vi "FPGA Acquire Loop.vi"(8 "error in (no error)":errorcluster, 10 "FIFO Buffers":refnum<k33>[](array[refnum]), 11 "Refnum in":refnum<k20>) -> ()   [LabVIEW 2014]
uses:
  Controls/RT Stream Data.ctl
  RT Stop.vi
  RT Tags.vi
  RT Comm Refs.vi
  <vilib>/Utility/error.llb/Error Cluster From Error Code.vi
  <vilib>/rvi/errors/niLvFpgaAdjustHostInterfaceError.vi
  <vilib>/rvi/interface/nirviMethod/nirviMethod.xnode
  <vilib>/rvi/interface/nirviReadWriteControl/nirviReadWriteControl.xnode
  <vilib>/FPGAPlugInAG/Dynamic/niLvFpga_ReadFifo_Dynamic.vi
  <vilib>/rvi/errors/niLvFpgaMergeErrorWithErrorCode.vi
  NiFpgaLv.dll
  <vilib>/rvi/interface/Simulation/niFpgaSimulationCallBeginRW.vi
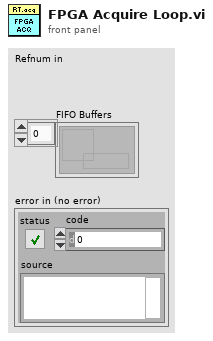
[diagram p1: front panel]
types:
  T1 = typedef "RT Stream Data.ctl" = cluster{"Temp Data":dbl[], "pH Data":dbl[]}
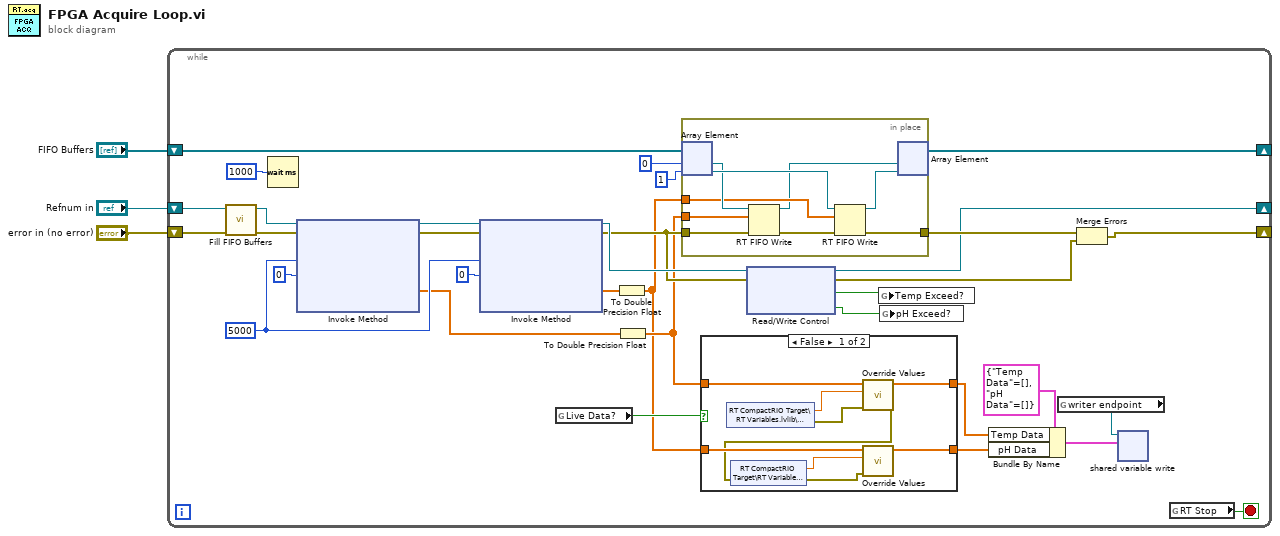
[diagram p0: block diagram]
diagram:
  n1 = while {
    shift-right: [w18] -> _
    shift-left: "Refnum in" -> [w36]
    shift-right: [w16] -> _
    shift-left: "error in (no error)" -> [w34]
    shift-right: [w21] -> _
    shift-left: "FIFO Buffers" -> [w26]
    stop <- w14 stop-if-true
    w30 = u32 5000 ("Number of Elements")
    n2 = call "Fill FIFO Buffers.vi"("error in (no error)"=w34, "Refnum in"=w36) -> ("error out"=w29:errorcluster, "Refnum out"=w33:refnum<k20>)  [unwired: 8 in]
    n3 = Wait (ms)(milliseconds to wait=u32 1000) -> ()  [unwired: 1 out]
    n4 = xnode "Invoke Method"("FPGA VI Reference In"=w33, "error in"=w29, "Number of Elements"=w30, "Timeout (ms)"=0) -> ("FPGA VI Reference Out"=w32:refnum<k20>, "error out"=w31:errorcluster, "Data"=w23:sgl[])  [unwired: 1 out]
    n5 = xnode "Invoke Method"("FPGA VI Reference In"=w32, "error in"=w31, "Number of Elements"=w30, "Timeout (ms)"=0) -> ("FPGA VI Reference Out"=w19:refnum<k20>, "error out"=w17:errorcluster, "Data"=w22:sgl[])  [unwired: 1 out]
    n6 = global read "RT Tags.vi" "Live Data?"() -> (w13:bool)
    n7 = To Double Precision Float(number=w22) -> (double precision float=w9:dbl[])
    n8 = To Double Precision Float(number=w23) -> (double precision float=w10:dbl[])
    n9 = in-place {
      in-place-border: w17 -> [w55]
      in-place-border: w10 -> [w52]
      in-place-border: w9 -> [w51]
      in-place-border: [w48] -> w20
      n10 = in-place-array #1(w26, 0, 1) -> (w53:refnum<k33>, w54:refnum<k33>)
      n11 = RT FIFO Write(0:w53, 1:w52, 3:w55) -> (8:w50:refnum<k33>, 11:w56:errorcluster)  [unwired: 2 in, 2 out]
      n12 = RT FIFO Write(0:w54, 1:w51, 3:w56) -> (8:w49:refnum<k33>, 11:w48:errorcluster)  [unwired: 2 in, 2 out]
      n13 = in-place-array #1(w50, w49) -> (w21:refnum<k33>[])  [unwired: 2 out]
    }
    n14 = case shown="False" w13 {
      tunnel: w10 -> [w45 w47]
      tunnel: w9 -> [w43 w46]
      tunnel: [w44 w47] -> w8
      tunnel: [w42 w46] -> w7
      frame False {
        n15 = shared-variable "RT CompactRIO Target\\RT Variables.lvlib\\TempOV"() -> (w41:dbl, error out=w39:errorcluster)  [unwired: 1 in]
        n16 = call "Override Values.vi"("error in (no error)"=w39, "Double"=w41, "Array in"=w45) -> ("error out"=w38:errorcluster, "Array out"=w44:dbl[])  [unwired: 7 in]
        n17 = shared-variable "RT CompactRIO Target\\RT Variables.lvlib\\pHOV"(error in=w38) -> (w40:dbl, error out=w37:errorcluster)
        n18 = call "Override Values.vi"("error in (no error)"=w37, "Double"=w40, "Array in"=w43) -> ("Array out"=w42:dbl[])  [unwired: 7 in, 1 out]
      }
      frame True {
      }
    }
    n19 = xnode "Read/Write Control"("FPGA VI Reference In"=w19, "error in"=w17) -> ("FPGA VI Reference Out"=w18:refnum<k20>, "error out"=w15:errorcluster, "Temp Exceed?"=w12:bool, "pH Exceed?"=w11:bool)
    n20 = global write "RT Tags.vi" "Temp Exceed?"(w12) -> ()
    n21 = global write "RT Tags.vi" "pH Exceed?"(w11) -> ()
    n22 = Bundle By Name(cluster=T1 {"Temp Data"=[], "pH Data"=[]}, "Temp Data"=w8, "pH Data"=w7) -> (w5:T1)
    n23 = global read "RT Comm Refs.vi" "writer endpoint"() -> (w4:refnum<k21>)
    n24 = Merge Errors(w20, w15) -> (w16:errorcluster)
    n25 = shared-variable-write(w4, w5) -> ()  [unwired: 2 in, 3 out]
    n26 = global read "RT Stop.vi" "RT Stop"() -> (w14:bool)
  }
